vi "Test DMA.vi"() -> ()   [LabVIEW 2014]
uses:
  DMA.lvclass
  DMA.lvclass/DMA.ctl
  Particle Class/Particle Properties.lvclass/Particle Properties.ctl
  Atmospheric/Gas Properties/Gas Properties.lvclass/Gas Properties.ctl
  Accessors/Write Qex.vi
  Accessors/Write Qsh.vi
  Accessors/Read Particle.vi
  Particle Class/Accessors/Write D.vi
  Accessors/Write Particle.vi
  Accessors/Read Gas Ref.vi
  Atmospheric/Gas Properties/Accessors/Write P (mb).vi
  Atmospheric/Gas Properties/Accessors/Write T (K).vi
  Accessors/Write Gas Ref.vi
  Conversion Constants.vi
  Get Voltage.vi
  Particle Class/Particle Properties.lvclass
  Atmospheric/Gas Properties/Gas Properties.lvclass
panel:
  out "Electric Mobility":dbl
  in  "P (mb)":dbl
  in  "T (degC)":dbl
  out "V":dbl
  in  "Dp (nm)":dbl
  in  "Qsh":dbl
  in  "Qex":dbl
  out "error out":errorcluster
  in  "Enum":T1(ring)
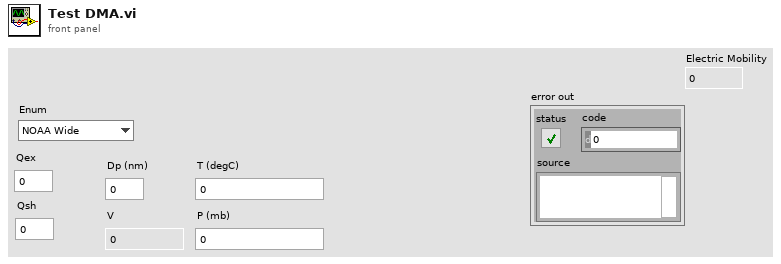
[diagram p1: front panel]
types:
  T1 = enum16{"NOAA Wide", "TSI 3071", "TSI 3081 Long", "TSI 3085 Nano", "GMW"}
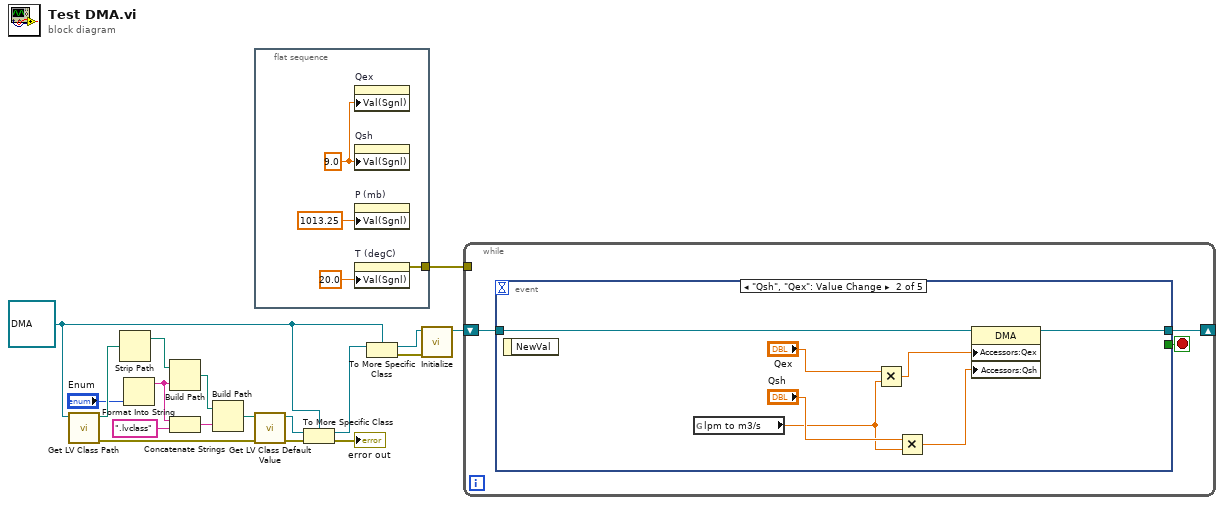
[diagram p0: block diagram]
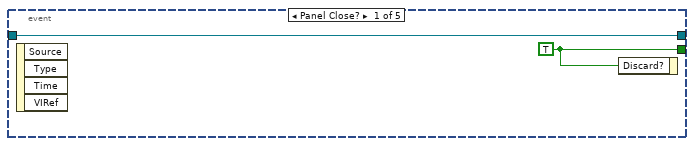
[diagram p2: hidden frame]
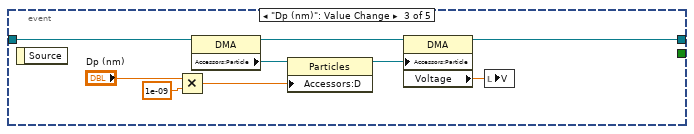
[diagram p3: hidden frame]
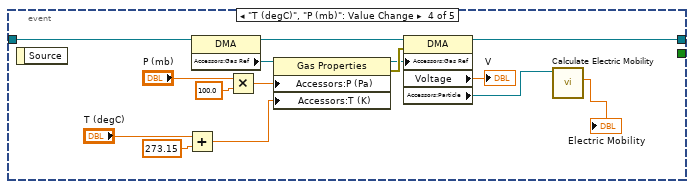
[diagram p4: hidden frame]
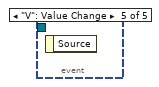
[diagram p5: hidden frame]
diagram:
  w5 = refnum<class "DMA.lvclass"> refnum ("DMA")
  n1 = call <vilib>:"Get LV Class Path.vi"("object"=w5) -> ("error out"=w10:errorcluster, "class path"=w18:path)  [unwired: 9 in]
  n2 = Strip Path(path=w18) -> (stripped path=w17:path)  [unwired: 1 out]
  n3 = Format Into String("Enum") -> (resulting string=w7:string)  [unwired: 3 in, 1 out]
  n4 = Build Path(base path=w17, name or relative path=w7) -> (appended path=w16:path)
  n5 = Concatenate Strings(w7, ".lvclass" ("string")) -> (w14:string)
  n6 = Build Path(base path=w16, name or relative path=w14) -> (appended path=w13:path)
  n7 = flat-sequence {
    tunnel: [w19] -> w1
    frame #0 {
      w22 = 9.0 ("Value (Signaling)")
      n8 = property on="Qex" class="DigNum (strict)"("Val(Sgnl)"=w22) -> ()  [unwired: 2 in, 2 out]
      n9 = property on="Qsh" class="DigNum (strict)"("Val(Sgnl)"=w22) -> ()  [unwired: 2 in, 2 out]
      n10 = property on="P (mb)" class="DigNum (strict)"("Val(Sgnl)"=1013.25 ("Value (Signaling)")) -> ()  [unwired: 2 in, 2 out]
      n11 = property on="T (degC)" class="DigNum (strict)"("Val(Sgnl)"=20.0 ("Value (Signaling)")) -> (error out=w19:errorcluster)  [unwired: 2 in, 1 out]
    }
  }
  n12 = call <vilib>:"Get LV Class Default Value.vi"("error in (no error)"=w10, "class path"=w13) -> ("error out"=w11:errorcluster, "object"=w12:refnum<class>)  [unwired: 8 in]
  n13 = To More Specific Class(target class=w5, reference=w12, error in=w11) -> (specific class reference=w6:refnum<class "DMA.lvclass">, error out=→"error out":errorcluster)
  n14 = To More Specific Class(target class=w5, reference=w6) -> (specific class reference=w4:refnum<class "DMA.lvclass">, error out=w3:errorcluster)  [unwired: 1 in]
  n15 = call-dynamic "Initialize.vi"("error in"=w3, "DMA in"=w4) -> ("DMA out"=w2:refnum<class "DMA.lvclass">)  [unwired: 8 in, 1 out]
  n16 = while {
    shift-right: [w23] -> _
    shift-left: w2 -> [w25]
    tunnel: w1 -> [_]
    stop <- w24 stop-if-true
    n17 = event shown="[1] \"Qsh\", \"Qex\": Value Change" {
      selector: _ -> [_ _ _ _ _]
      dyn-events: _ -> [_ _ _ _ _]
      timeout: _ -> [_ _ _ _ _]
      tunnel: w25 -> [w26 w34 w43 w58 _]
      tunnel: [w27 _ _ _ _] -> w24
      tunnel: [w26 w33 w35 w53 _] -> w23
      event Panel Close? {
        w27 = TRUE ("Discard?")
        n18 = event-data() -> ()  [unwired: 1 in, 4 out]
        n19 = event-data("Discard?"=w27) -> ()  [unwired: 1 in, 1 out]
      }
      event "Qsh", "Qex": Value Change {
        n20 = event-data() -> ()  [unwired: 1 in, 1 out]
        n21 = global read "Conversion Constants.vi" "lpm to m3/s"() -> (w30:dbl)
        n22 = Multiply(x="Qex", y=w30) -> (x*y=w28:dbl)
        n23 = Multiply(x="Qsh", y=w30) -> (x*y=w29:dbl)
        n24 = property class="DMA"(reference=w34, "Accessors:Qex"=w28, "Accessors:Qsh"=w29) -> (reference out=w33:refnum<class "DMA.lvclass">)  [unwired: 1 in, 1 out]
      }
      event "Dp (nm)": Value Change {
        n25 = event-data() -> ()  [unwired: 1 in, 1 out]
        n26 = Multiply(x="Dp (nm)", y=1e-09) -> (x*y=w39:dbl)
        n27 = property class="DMA"(reference=w43) -> (reference out=w38:refnum<class "DMA.lvclass">, "Accessors:Particle"=w42:refnum<class "Particle Properties.lvclass">)  [unwired: 1 in, 1 out]
        n28 = property class="Particles"(reference=w42, "Accessors:D"=w39) -> (reference out=w37:refnum<class "Particle Properties.lvclass">)  [unwired: 1 in, 1 out]
        n29 = property class="DMA"(reference=w38, "Accessors:Particle"=w37) -> (reference out=w35:refnum<class "DMA.lvclass">, "Voltage"=w36:dbl)  [unwired: 1 in, 1 out]
        n30 = local write "V"(w36) -> ()
      }
      event "T (degC)", "P (mb)": Value Change {
        n31 = event-data() -> ()  [unwired: 1 in, 1 out]
        n32 = Add(x="T (degC)", y=273.15) -> (x+y=w47:dbl)
        n33 = property class="DMA"(reference=w58) -> (reference out=w56:refnum<class "DMA.lvclass">, "Accessors:Gas Ref"=w57:refnum<data-value>)  [unwired: 1 in, 1 out]
        n34 = Multiply(x="P (mb)", y=100.0) -> (x*y=w50:dbl)
        n35 = property class="Gas Properties"(reference=w57, "Accessors:P (Pa)"=w50, "Accessors:T (K)"=w47) -> (reference out=w54:refnum<data-value>, error out=w55:errorcluster)  [unwired: 1 in]
        n36 = property class="DMA"(reference=w56, error in=w55, "Accessors:Gas Ref"=w54) -> (reference out=w53:refnum<class "DMA.lvclass">, "Voltage"=→"V":dbl, "Accessors:Particle"=w45:refnum<class "Particle Properties.lvclass">)  [unwired: 1 out]
        n37 = call "Calculate Electric Mobility.vi"("Particles in"=w45) -> ("Z"=→"Electric Mobility":dbl)  [unwired: 8 in, 2 out]
      }
      event "V": Value Change {
        n38 = event-data() -> ()  [unwired: 1 in, 1 out]
      }
    }
  }
